vi "ws_configure Standalone Stop.vi"(4 "error in (no error)":errorcluster) -> (0 "error out":errorcluster)   [LabVIEW 2011]
doc: "Programmatically tests the state of the HTTP Server. This VI also can load and start, or stop and unload the server VIs."
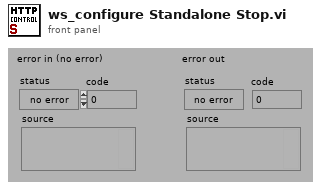
[diagram p1: front panel]
types:
  T1 = enum32{"Bad", "Idle", "Run top level", "Running"}
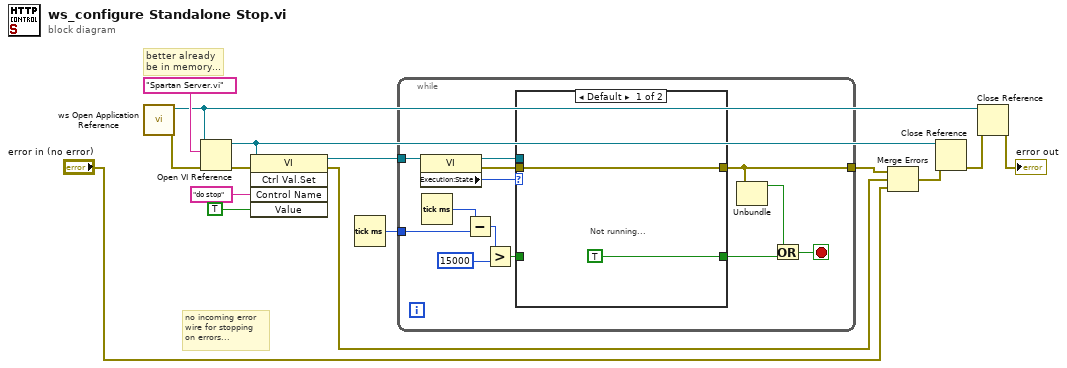
[diagram p0: block diagram]
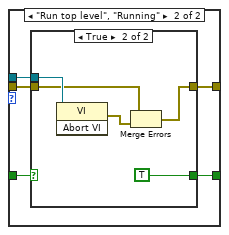
[diagram p2: hidden frame]
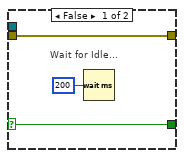
[diagram p3: hidden frame]
diagram:
  # "better already\nbe in memory..."
  # "no incoming error\nwire for stopping\non errors..."
  n1 = call "ws Open Application Reference.vi"() -> ("error out"=w1:errorcluster, "application reference"=w2:refnum<vi>)  [unwired: 10 in]
  n2 = Open VI Reference(application reference (local)=w2, vi path="Spartan Server.vi", error in (no error)=w1) -> (vi reference=w5:refnum<vi>, error out=w12:errorcluster)  [unwired: 3 out]
  n3 = invoke class="VI" method="Ctrl Val.Set"(reference=w5, error in=w12, "Control Name"="do stop", "Value"=TRUE) -> (reference out=w8:refnum<vi>, error out=w6:errorcluster)  [unwired: 1 in, 3 out]
  n4 = Tick Count (ms)() -> (millisecond timer value=w11:u32)
  n5 = while {
    tunnel: w8 -> [w28]
    tunnel: w11 -> [w25]
    tunnel: [w17] -> w10
    stop <- w21 stop-if-true
    n6 = property class="VI"(reference=w28) -> (reference out=w18:refnum<vi>, error out=w19:errorcluster, "Execution:State"=w27:T1)  [unwired: 1 in]
    n7 = Tick Count (ms)() -> (millisecond timer value=w26:u32)
    n8 = Subtract(x=w26, y=w25) -> (x-y=w24:u32)
    n9 = Greater?(x=w24, y=u32 15000 ("Timeout (15000)")) -> (0:w20:bool)
    n10 = case shown="Default" w27 {
      tunnel: [TRUE w32] -> w22
      tunnel: w20 -> [_ w35]
      tunnel: w19 -> [w29 w34]
      tunnel: [w29 w33] -> w17
      tunnel: w18 -> [_ w31]
      frame Default {
        # "Not running..."
      }
      frame "Run top level", "Running" {
        n11 = case shown="True" w35 {
          selector: w35 -> [w36 _]
          tunnel: w34 -> [w37 w42]
          tunnel: [w37 w40] -> w33
          tunnel: [w36 TRUE] -> w32
          tunnel: w31 -> [_ w43]
          frame False {
            # "Wait for Idle..."
            n12 = Wait (ms)(milliseconds to wait=u32 200) -> ()  [unwired: 1 out]
          }
          frame True {
            n13 = invoke class="VI" method="Abort VI"(reference=w43) -> (error out=w41:errorcluster)  [unwired: 2 in, 2 out]
            n14 = Merge Errors(w42, w41) -> (w40:errorcluster)
          }
        }
      }
    }
    n15 = Unbundle(w17) -> ("status"=w23:bool)  [unwired: 2 out]
    n16 = Or(x=w23, y=w22) -> (x .or. y?=w21:bool)
  }
  n17 = Merge Errors(w10, w6, "error in (no error)") -> (w9:errorcluster)
  n18 = Close Reference(reference=w5, error in (no error)=w9) -> (error out=w4:errorcluster)
  n19 = Close Reference(reference=w2, error in (no error)=w4) -> (error out=→"error out":errorcluster)
